vi "GdsLanguage_GetAttributes.vi"(5 "error in (no error)":errorcluster) -> (16 "Attributes":T1, 19 "error out":errorcluster)   [LabVIEW 2014]
doc: "Returns the attributes of a AcTranslator or subclass object.\n\nIf the object is currently locked for modification, 'Attibutes locked?' will return TRUE.\n\n[GOOP 2.0.13]"
uses:
  <resource>/Framework/Providers/Open_GDS/ClassProviders/Common/GdsLanguage/private/GdsLanguage_ObjectAttributes.ctl
  <resource>/Framework/Providers/Open_GDS/ClassProviders/Common/GdsLanguage/GdsLanguage_LanguageID.ctl
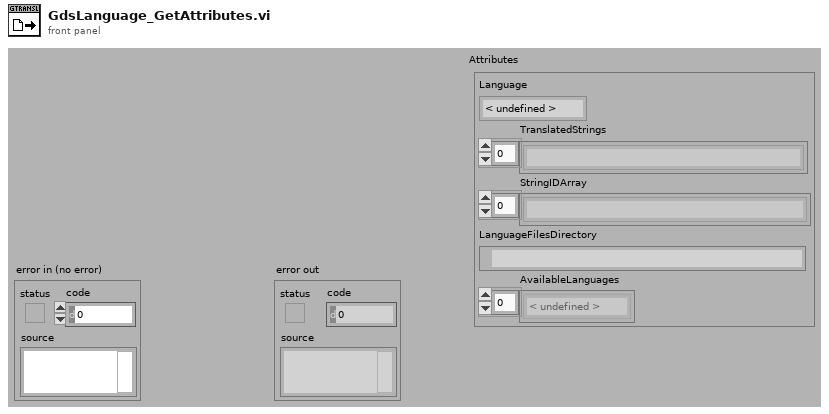
[diagram p1: front panel]
types:
  T1 = typedef "GdsLanguage_ObjectAttributes.ctl" = cluster{"Language":T2, "TranslatedStrings":string[], "StringIDArray":string[], "LanguageFilesDirectory":path, "AvailableLanguages":T2[]}
  T2 = typedef "GdsLanguage_LanguageID.ctl" = enum16{"< undefined >", "aa", "ab", "af", "am", "ar", "as", "ay", "az", "ba", "be", "bg", "bh", "bi", "bn", "bo", "br", "ca", "co", "cs", "cy", "da", "de", "dz", "el", "en", "eo", "es", "et", "eu", "fa", "fi", "fj", "fo", "fr", "fy", "ga", "gd", "gl", "gn", "gu", "gv", "ha", "he", "hi", "hr", "hu", "hy", "ia", "id", "ie", "ik", "is", "it", "iu", "ja", "jv", "ka", "kk", "kl", "km", "kn", "ko", "ks", "ku", "ky", "la", "li", "ln", "lo", "lt", "lv", "mg", "mi", "mk", "ml", "mn", "mo", "mr", "ms", "mt", "my", "na", "ne", "nl", "no", "oc", "om", "or", "pa", "pl", "ps", "pt", "qu", "rm", "rn", "ro", "ru", "rw", "sa", "sd", "sg", "sh", "si", "sk", "sl", "sm", "sn", "so", "sq", "sr", "ss", "st", "su", "sv", "sw", "ta", "te", "tg", "th", "ti", "tk", "tl", "tn", "to", "tr", "ts", "tt", "tw", "ug", "uk", "ur", "uz", "vi", "vo", "wo", "xh", "yi", "yo", "zh", "zu"}
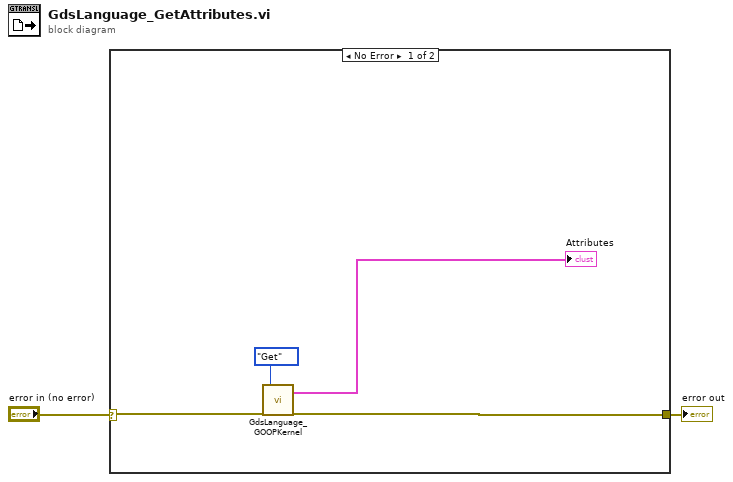
[diagram p0: block diagram]
diagram:
  n1 = case shown="No Error" "error in (no error)" {
    selector: "error in (no error)" -> [w6 w7]
    tunnel: [w5 w7] -> w2
    frame No Error {
      n2 = call <resource>:"GdsLanguage_GOOPKernel.vi"("error in (no error)"=w6, "Action"=enum16{"Get", "Set"}."Get") -> ("Data out"=→"Attributes":T1, "error out"=w5:errorcluster)  [unwired: 16 in]
    }
    frame Error {
    }
  }
  "error out" <- w2
